vi "TestModule.vi"   [LabVIEW 2025, in "PLC_Module.lvlib"]
uses:
  PLC_Module.lvlib
  PLC_Module/PLC_Module.lvclass
  Msg.ctl
  PLC_Module/PLC_Type.ctl
  PLC_Module/PLC_Module.lvclass/PLC_Module.ctl
  PLC_Module Messages/SendActorCoreMsg Msg/SendActorCoreMsg Msg.lvclass/SendActorCoreMsg Msg.ctl
  <vilib>/ActorFramework/Message Enqueuer/Message Enqueuer.lvclass/Message Enqueuer.ctl
  PLC_Module Messages/Connection Msg/Connection Msg.lvclass/Connection Msg.ctl
  19cab44c-1e26-4b9c-8ac8-9b8d5054e390.vi
  PLC_Module/Write Type.vi
  PLC_Module/Write Debug.vi
  PLC_Module/Write ModuleName.vi
  <vilib>/ActorFramework/Message Enqueuer/Enqueue.vi
  PLC_Module Messages/SendActorCoreMsg Msg/SendActorCoreMsg Msg.lvclass
  PLC_Module Messages/Connection Msg/Connection Msg.lvclass
  <vilib>/ActorFramework/Message Priority Queue/Priority Enqueue.vi
  <vilib>/ActorFramework/Actor/Actor.lvclass
types:
  T1 = typedef "PLC_Module.lvlib/PLC_Module.lvclass/PLC_Type.ctl" = enum16{"Simulated_PLC", "SIMATIC_S7"}
  T2 = typedef "Msg.ctl" = string
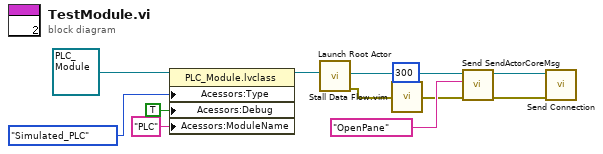
[diagram p0: block diagram]
diagram:
  n1 = property class="PLC_Module.lvclass"(reference=refnum<class "PLC_Module.lvclass"> refnum ("PLC_Module.lvlib:PLC_Module.lvclass"), "Acessors:Type"=PLC_Type."Simulated_PLC" ("Type"), "Acessors:Debug"=TRUE ("Debug"), "Acessors:ModuleName"="PLC" ("ModuleName")) -> (reference out=w9:refnum<class "PLC_Module.lvclass">)  [unwired: 1 in, 1 out]
  n2 = call <vilib>:"Launch Root Actor.vi"("Actor"=w9) -> ("error out"=w6:errorcluster, "Actor's Enqueuer"=w11:refnum<class "Message Enqueuer.lvclass">)  [unwired: 9 in]
  n3 = call "Stall Data Flow.vim"("value in"=w6, "milliseconds to wait"=u32 300) -> ("value out"=w5:errorcluster)  [unwired: 1 out]
  n4 = call "Send SendActorCoreMsg.vi"("error in (no error)"=w5, "Msg"=T2 "OpenPane", "Message Enqueuer"=w11) -> ("error out"=w1:errorcluster, "Message Enqueuer out"=w2:refnum<class "Message Enqueuer.lvclass">)  [unwired: 7 in]
  n5 = call "Send Connection.vi"("error in (no error)"=w1, "Message Enqueuer"=w2) -> ()  [unwired: 7 in, 3 out]
